vi "Initialize Console Options.vi"(8 "error in (no error)":errorcluster, 11 "Normal Entry Console View in":refnum<class "Normal Entry Console View.lvclass">) -> (0 "error out":errorcluster, 3 "Normal Entry Console View out":refnum<class "Normal Entry Console View.lvclass">)   [LabVIEW 2019, in "Normal Entry Console View.lvclass"]
uses:
  <vilib>/gpm_packages/@cs/Car-wash/Source/Normal Entry Console View/Normal Entry Console View/Normal Entry Console View.lvclass
  C:/Program Files/National Instruments/LabVIEW 2019/vi.lib/gpm_packages/@cs/Car-wash/Source/Entry Console View Definition/Entry Console View Definition/Entry Console View Definition.lvclass
  <vilib>/gpm_packages/@cs/Car-wash/Source/Entry Console View Definition/Entry Console View Definition/Entry Console View Definition.lvclass
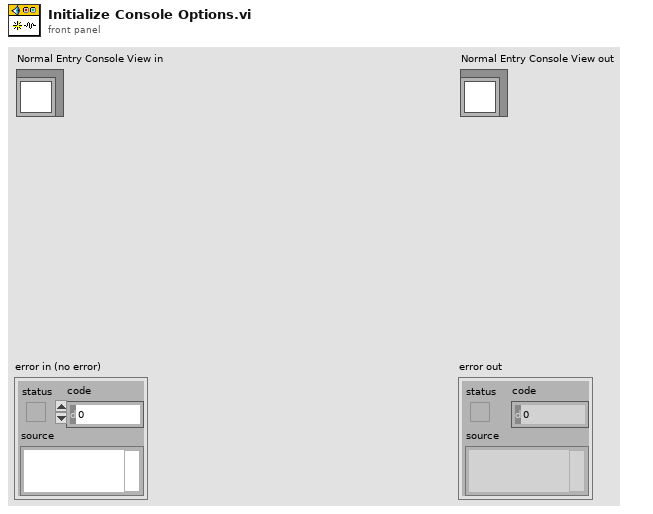
[diagram p1: front panel]
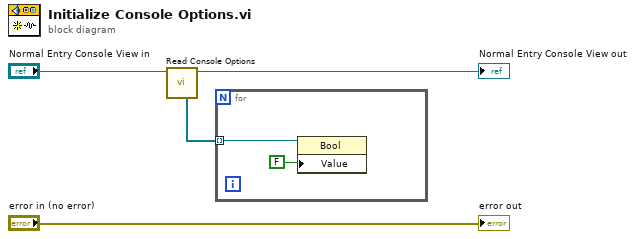
[diagram p0: block diagram]
diagram:
  n1 = call <vilib>:"Read Console Options.vi"("Entry Console View Definition in"="Normal Entry Console View in") -> ("Entry Console View Definition out"=→"Normal Entry Console View out":refnum<class "Normal Entry Console View.lvclass">, "Console Options"=w3:refnum<vi>[])  [unwired: 9 in]
  n2 = for {
    tunnel: w3 -> [w6] mode=indexing
    n3 = property class="Bool"(reference=w6, "Value"=FALSE) -> ()  [unwired: 1 in, 2 out]
  }
  "error out" <- "error in (no error)"
